vi "updateScale.vi"(8 "error in (no error)":errorcluster, 10 "firstImage?":bool, 11 "ImageStreamViewer in":refnum<class "ImageStreamViewer.lvclass">) -> (0 "error out":errorcluster, 3 "ImageStreamViewer out":refnum<class "ImageStreamViewer.lvclass">)   [LabVIEW 2011, in "Views.lvlib" / "Camera.lvlib" / "ImageStreamViewer.lvclass"]
uses:
  ImageStreamViewer.lvclass
  ImageStreamViewer.lvclass/ImageStreamViewer.ctl
  <vilib>/vision/NI_Vision_Development_Module.lvlib
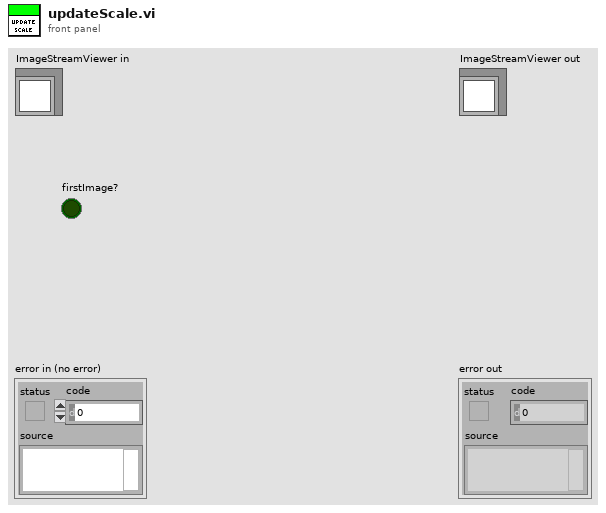
[diagram p1: front panel]
types:
  T1 = typedef "IMAQ Image.ctl" = refnum<image>
  T2 = cluster{"histogram":u32[], "Minimal Value":sgl, "Maximal Value":sgl, "Starting Value":sgl, "Interval Width":sgl, "Mean Value":sgl, "Standard  Variation":sgl, "Area (pixels)":i32}
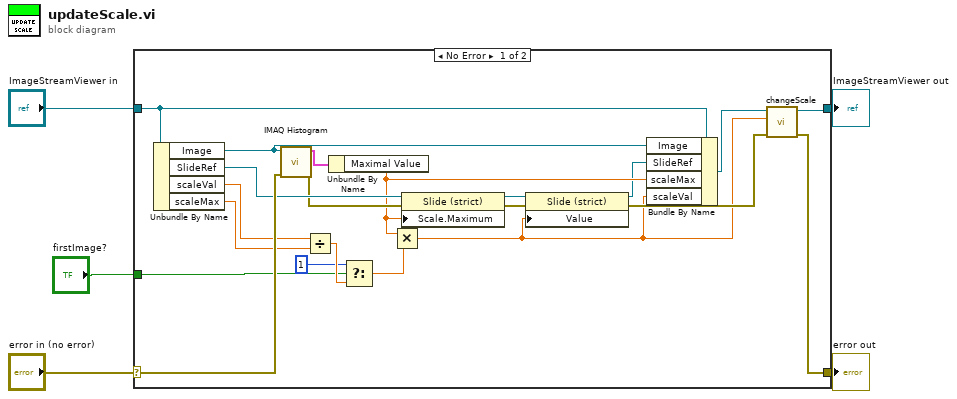
[diagram p0: block diagram]
diagram:
  n1 = case shown="No Error" "error in (no error)" {
    selector: "error in (no error)" -> [w26 w28]
    tunnel: [w18 w28] -> w4
    tunnel: [w19 w27] -> w2
    tunnel: "ImageStreamViewer in" -> [w22 w27]
    tunnel: "firstImage?" -> [w8 _]
    frame No Error {
      n2 = Unbundle By Name(w22) -> ("Image"=w21:T1, "SlideRef"=w24:refnum<vi>, "scaleVal"=w7:dbl, "scaleMax"=w17:dbl)
      n3 = call "IMAQ Histogram"("error in (no error)"=w26, "Image"=w21) -> ("error out"=w23:errorcluster, "Histogram Report"=w25:T2)  [unwired: 8 in]
      n4 = Divide(x=w7, y=w17) -> (x/y=w11:dbl)
      n5 = Unbundle By Name(w25) -> ("Maximal Value"=w16:sgl)
      n6 = Select(t=1, s=w8, f=w11) -> (s? t:f=w9:dbl)
      n7 = Multiply(x=w16, y=w9) -> (x*y=w6:dbl)
      n8 = property class="Slide (strict)"(reference=w24, error in=w23, "Scale.Maximum"=w16) -> (reference out=w15:refnum<vi>, error out=w14:errorcluster)
      n9 = property class="Slide (strict)"(reference=w15, error in=w14, "Value"=w6) -> (reference out=w13:refnum<vi>, error out=w12:errorcluster)
      n10 = Bundle By Name(cluster=w22, "Image"=w21, "SlideRef"=w13, "scaleMax"=w16, "scaleVal"=w6) -> (w20:refnum<class "ImageStreamViewer.lvclass">)
      n11 = call "changeScale.vi"("error in (no error)"=w12, "newValue"=w6, "ImageStreamViewer in"=w20) -> ("error out"=w18:errorcluster, "ImageStreamViewer out"=w19:refnum<class "ImageStreamViewer.lvclass">)  [unwired: 7 in]
    }
    frame Error {
    }
  }
  "error out" <- w4
  "ImageStreamViewer out" <- w2
